vi "Set Disabled.vi"(8 "error in (no error)":errorcluster, 10 "Disabled":bool, 11 "GaugeIndicator in":refnum<class "GaugeIndicator.lvclass">) -> (0 "error out":errorcluster, 3 "GaugeIndicator out":refnum<class "GaugeIndicator.lvclass">)   [LabVIEW 2020, in "VolatusGUIElements.lvlib" / "GaugeIndicator.lvclass"]
uses:
  GaugeIndicator.lvclass
  GaugeIndicator.lvclass/GaugeIndicator.ctl
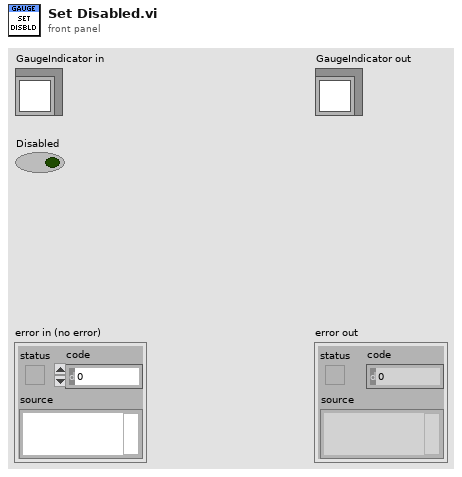
[diagram p1: front panel]
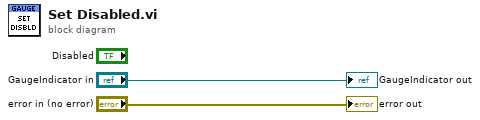
[diagram p0: block diagram]
diagram:
  "error out" <- "error in (no error)"
  "GaugeIndicator out" <- "GaugeIndicator in"
